vi "Update Open Thermocouple Status Table.vi"(0 "Open Thermocouple Status Table":refnum<vi>, 5 "Open Thermocouple Channels":string[](array[string]), 7 "Task Channels":refnum<k21>[](array[refnum]), 9 "Cumulative Status In":bool[](array[boolean]), 11 "Error In":errorcluster) -> (10 "Cumulative Status Out":bool[](array[boolean]), 15 "Error Out":errorcluster)   [LabVIEW 2022 SP3]
doc: "This VI converts the current open thermocouple status and cumulative open thermocouple status into a table displaying the status as \"Normal\" or \"Open\"."
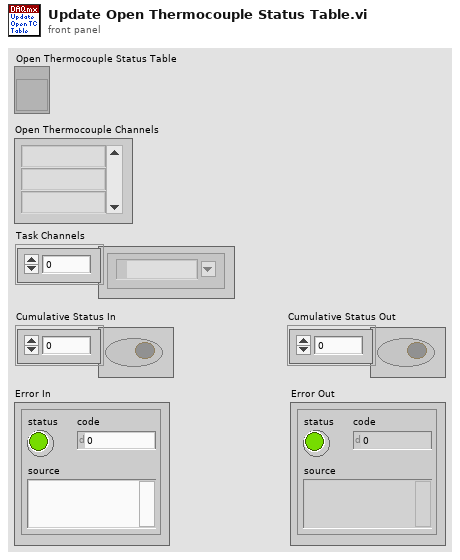
[diagram p1: front panel]
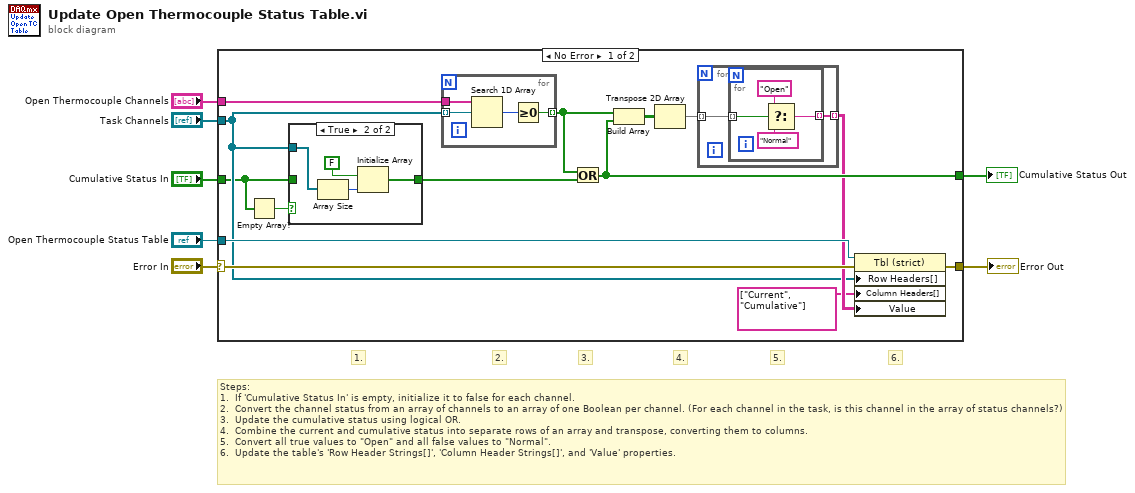
[diagram p0: block diagram]
diagram:
  # "6."
  # "5."
  # "4."
  # "3."
  # "2."
  # "1."
  # "Steps:\n1.  If 'Cumulative Status In' is empty, initialize it to false for each channel.\n2.  Convert the channel status from an array of channels to an array of one Boolean per channel. (For each channel in the task, is this channel in the array of status channels?)\n3.  Update the cumulative status using logical OR.\n4.  Combine the current and cumulative status into separate rows of an array and transpose, converting them to columns.\n5.  Convert all true values to \"Open\" and all false values to \"Normal\".\n6.  Update the table's 'Row Header Strings[]', 'Column Header Strings[]', and 'Value' properties."
  n1 = case shown="No Error" "Error In" {
    selector: "Error In" -> [w17 w38]
    tunnel: [w21 w37] -> w3
    tunnel: "Cumulative Status In" -> [w9 w37]
    tunnel: "Task Channels" -> [w13 _]
    tunnel: "Open Thermocouple Channels" -> [w12 _]
    tunnel: [w15 w38] -> w5
    tunnel: "Open Thermocouple Status Table" -> [w16 _]
    frame No Error {
      n2 = Empty Array?(array=w9) -> (empty?=w8:bool)
      n3 = case shown="True" w8 {
        tunnel: w9 -> [w26 _]
        tunnel: [w26 w28] -> w18
        tunnel: w13 -> [_ w27]
        frame False {
        }
        frame True {
          n4 = Array Size(array=w27) -> (size(s)=w29:i32)
          n5 = Initialize Array(FALSE, w29) -> (w28:bool[])
        }
      }
      n6 = for {
        tunnel: [w24] -> w11 mode=indexing
        tunnel: w13 -> [w23] mode=indexing
        tunnel: w12 -> [w22]
        n7 = Search 1D Array(1D array=w22, element=w23) -> (index of element=w25:i32)  [unwired: 1 in]
        n8 = Greater Or Equal To 0?(x=w25) -> (x >= 0?=w24:bool)
      }
      n9 = Or(x=w11, y=w18) -> (x .or. y?=w21:bool[])
      n10 = Build Array(w11, w21) -> (w20:bool[][])
      n11 = Transpose 2D Array(2D array=w20) -> (transposed array=w19:bool[][])
      n12 = for {
        tunnel: [w32] -> w14 mode=indexing
        tunnel: w19 -> [w31] mode=indexing
        n13 = for {
          tunnel: [w36] -> w32 mode=indexing
          tunnel: w31 -> [w35] mode=indexing
          n14 = Select(t="Open" ("True String"), s=w35, f="Normal" ("False String")) -> (s? t:f=w36:string)
        }
      }
      n15 = property class="Tbl (strict)"(reference=w16, error in=w17, "Row Headers[]"=w13, "Column Headers[]"=string[] ["Current", "Cumulative"] ("Column Header Strings[]"), "Value"=w14) -> (error out=w15:errorcluster)  [unwired: 1 out]
    }
    frame Error {
    }
  }
  "Error Out" <- w5
  "Cumulative Status Out" <- w3
